vi "res_Get Resistance.vi"(8 "error in (no error)":errorcluster, 10 "Channel (1-10)":i8=1 min=1 max=66 step=1 format="%.1f", 11 "instrument handle":refnum<visa-resource-name>) -> (0 "error out":errorcluster, 1 "Actual Resistance":dbl, 2 "status":i32 format="%.0x", 3 "instrument handle out":refnum<visa-resource-name>)   [LabVIEW 2014, in "Pickering 40-295.lvlib"]
doc: "VI shows how to control resistor values on a 40-290 board\nthe example is using a 16 bit dual resistor chain 0...32k Ohm.\n\nThis example VI uses the pi40 VISA driver. Resistance values in 0.5 ohm steps can be entered (0.0 to 32767.5) in the \"Enter Resistance Value\" field. The appropriate bit will be set and relays closed. \n\nAn OFF LED indicates an open relay and a resistance value included in the resistance chain. An ON LED indicates a closed switch, a resistance value shorted out and not included in the resistance chain."
uses:
  Pickering 40-295.lvlib
panel:
  out "element":u32
  # "32768"
  # "16384"
  # "8192"
  # "4096"
  # "2048"
  # "1024"
  # "512"
  # "256"
  # "128"
  # "64"
  # "32"
  # "16"
  # "8"
  # "4"
  # "2"
  # "1"
  # "Max R   65535\nmin R 1 Ohm, 1 Ohm steps"
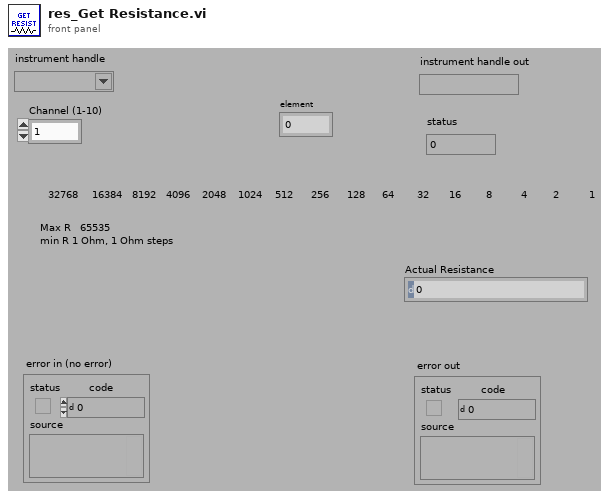
[diagram p1: front panel]
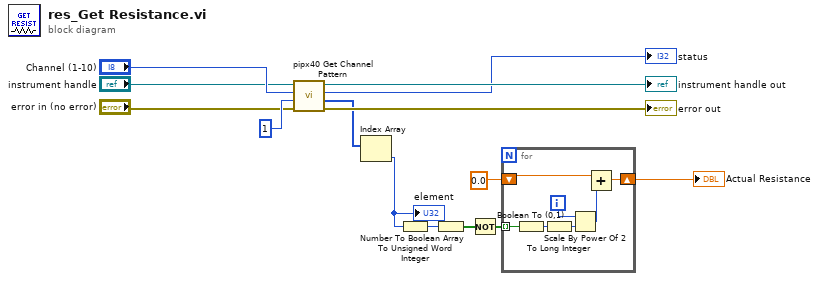
[diagram p0: block diagram]
diagram:
  n1 = call "pipx40 Get Channel Pattern.vi"("error in (no error)"="error in (no error)", "size of pattern"=u32 1, "subunit number"="Channel (1-10)", "instrument handle"="instrument handle") -> ("error out"=→"error out":errorcluster, "pattern"=w5:u32[], "status"=→"status":i32, "instrument handle out"=→"instrument handle out":refnum<visa-resource-name>)  [unwired: 4 out]
  n2 = Index Array(array=w5) -> (element=w4:u32)  [unwired: 1 in]
  "element" <- w4
  n3 = To Unsigned Word Integer(number=w4) -> (unsigned 16bit integer=w11:u16)
  n4 = Number To Boolean Array(number=w11) -> (Boolean array=w14:bool[])
  n5 = Not(x=w14) -> (.not. x?=w13:bool[])
  n6 = for {
    tunnel: w13 -> [w19] mode=indexing
    shift-right: [w16] -> w10
    shift-left: 0.0 -> [w17]
    i -> [w20]
    n7 = Boolean To (0,1)(Boolean=w19) -> (0, 1=w21:i16)
    n8 = To Long Integer(number=w21) -> (32bit integer=w15:i32)
    n9 = Scale By Power Of 2(n=w20, x=w15) -> (x*2^n=w18:i32)
    n10 = Add(x=w17, y=w18) -> (x+y=w16:dbl)
  }
  "Actual Resistance" <- w10
